vi "Plugin Options Panel End.vi"(6 "Index in":i32, 8 "error in (no error)":errorcluster, 9 "Config VI Refnum in":refnum<vi>, 10 "Container in":refnum<vi>, 11 "Plugins in":refnum<class "Plugin.lvclass">[](array[class])) -> (0 "error out":errorcluster, 2 "Container out":refnum<vi>, 3 "Plugins out":refnum<class "Plugin.lvclass">[](array[class]))   [LabVIEW 2015, in "Application.lvclass"]
uses:
  Application.lvclass
  Plugin.lvclass
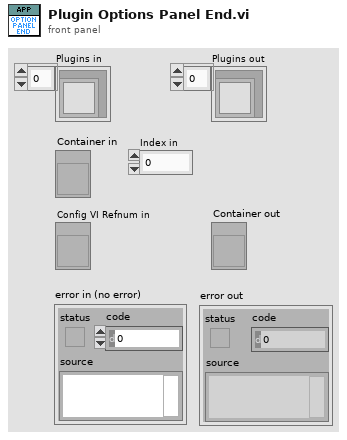
[diagram p1: front panel]
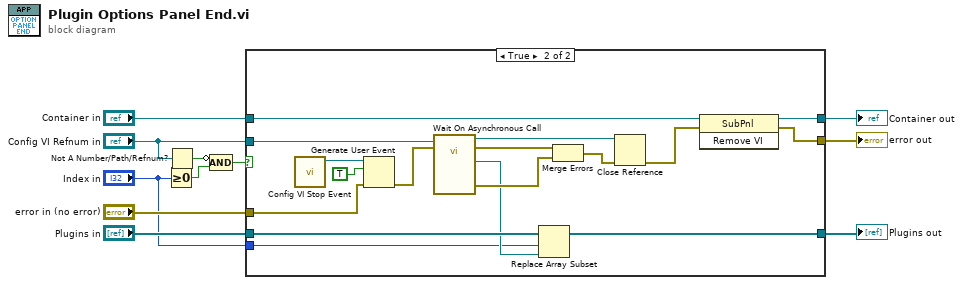
[diagram p0: block diagram]
diagram:
  n1 = Greater Or Equal To 0?(x="Index in") -> (x >= 0?=w3:bool)
  n2 = Not A Number/Path/Refnum?(number/path/refnum="Config VI Refnum in") -> (NaN/Path/Refnum?=w4:bool)
  n3 = Compound Arithmetic op=AND(invert w4, w3) -> (w2:bool)
  n4 = case shown="True" w2 {
    tunnel: "error in (no error)" -> [w13 w29]
    tunnel: "Container in" -> [w14 w23]
    tunnel: [w13 w21] -> w9
    tunnel: [w14 w20] -> w8
    tunnel: "Config VI Refnum in" -> [_ w19]
    tunnel: "Plugins in" -> [w12 w18]
    tunnel: [w12 w16] -> w5
    tunnel: "Index in" -> [_ w15]
    frame False {
    }
    frame True {
      n5 = call "Config VI Stop Event.vi"() -> ("VI Stop event"=w31:refnum<user-event>)  [unwired: 11 in]
      n6 = Generate User Event(user event=w31, event data cluster=TRUE, error in=w29) -> (error out=w28:errorcluster)  [unwired: 1 in, 1 out]
      n7 = call-by-ref "Wait On Asynchronous Call"(reference=w19, error in=w28) -> (reference out=w25:refnum<vi>, error out=w27:errorcluster, 0:"error out"=w26:errorcluster, "Plugin out"=w17:refnum<class "Plugin.lvclass">)  [unwired: 10 in]
      n8 = Replace Array Subset(array=w18, new element=w17, index=w15) -> (w16:refnum<class "Plugin.lvclass">[])
      n9 = Merge Errors(w27, w26) -> (w24:errorcluster)
      n10 = Close Reference(reference=w25, error in (no error)=w24) -> (error out=w22:errorcluster)
      n11 = invoke class="SubPnl" method="Remove VI"(reference=w23, error in=w22) -> (reference out=w20:refnum<vi>, error out=w21:errorcluster)  [unwired: 1 in, 1 out]
    }
  }
  "error out" <- w9
  "Container out" <- w8
  "Plugins out" <- w5
